vi "Write Waveform Number of Elements.vi"(10 "number of elements":u64, 11 "AO in":refnum<class "Analog Output.lvclass">) -> (3 "done":bool)   [LabVIEW 2017, in "Analog IO.lvlib" / "Analog Output.lvclass"]
uses:
  Analog Output.lvclass
  Analog Output.lvclass/Analog Output.ctl
  <vilib>/rvi/DataTransferAndStorage/Container/Common/niFpgaContainerExecOnDevCompGetState.vi
  <vilib>/rvi/Emulation/niFpgaEmulationIsFPGAContextNoSignature.vi
  <vilib>/rvi/DataTransferAndStorage/Container/Common/niFpgaContainerGetUniqueNameForEmu.vi
  <vilib>/rvi/eio/common/nirviEmuReportErrorAndStop.vi
  <vilib>/rvi/Emulation/niFpgaSctlEmulationGetInTimedLoop.vi
  <vilib>/rvi/Emulation/niFpgaProcessEmulError.vi
  <vilib>/rvi/DataTransferAndStorage/Container/XNode/niFpgaContainer.xnode
  <vilib>/rvi/DataTransferAndStorage/Handshake/Emulation/niFpgaHandshakeEmulationRefIn.vi
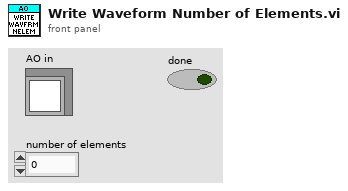
[diagram p1: front panel]
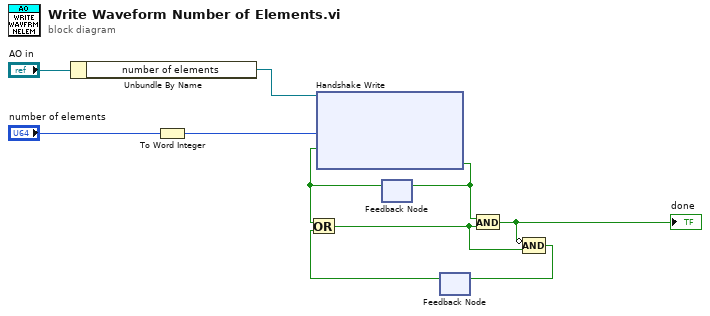
[diagram p0: block diagram]
diagram:
  n1 = Unbundle By Name("AO in") -> ("number of elements"=w6:refnum<k21>)
  n2 = To Word Integer(number="number of elements") -> (16bit integer=w3:i16)
  n3 = feedback #1() -> (w2:bool)  [unwired: 1 in]
  n4 = xnode ("Handshake Write")("Data"=w3, "Input Valid"=w2, "Handshake In"=w6) -> ("Ready for Input"=w1:bool)  [unwired: 1 out]
  n5 = feedback-in #1(w1) -> ()
  n6 = feedback #2() -> (w10:bool)  [unwired: 1 in]
  n7 = Or(x=w2, y=w10) -> (x .or. y?=w8:bool)
  n8 = And(x=w1, y=w8) -> (x .and. y?=w7:bool)
  "done" <- w7
  n9 = Compound Arithmetic op=AND(invert w7, w8) -> (w9:bool)
  n10 = feedback-in #2(w9) -> ()
